vi "StructureFactory.vi"(8 "error in":errorcluster, 11 "reference":refnum<vi>) -> (0 "error out":errorcluster, 3 "structure out":refnum<class "Structure.lvclass">)   [LabVIEW 2014, in "Raspberry Pi Compatible Compiler for LabVIEW.lvlib" / "Structure.lvclass"]
uses:
  Structure.lvclass
  CaseStructure/CaseStructure.lvclass
  Loop/Loop.lvclass
  DiagramDisable/DiagramDisable.lvclass
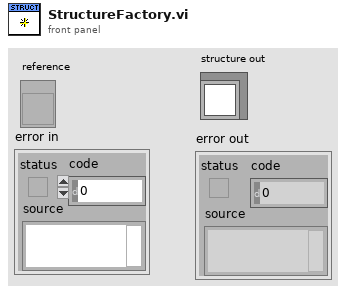
[diagram p1: front panel]
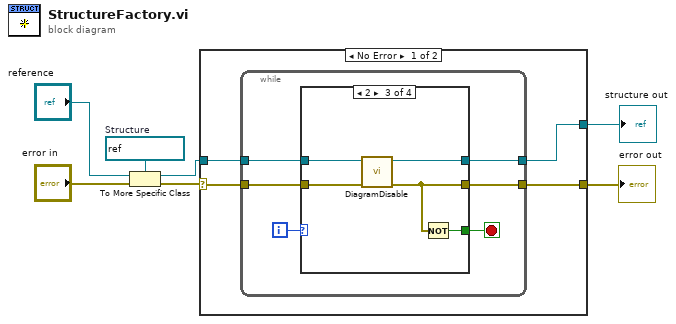
[diagram p0: block diagram]
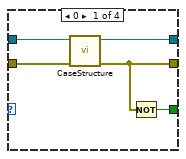
[diagram p2: hidden frame]
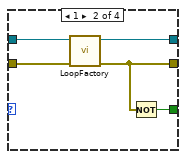
[diagram p3: hidden frame]
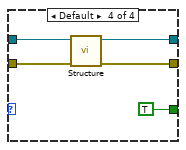
[diagram p4: hidden frame]
diagram:
  w7 = refnum<vi> refnum  # Structure
  n1 = To More Specific Class(target class=w7, reference="reference", error in="error in") -> (specific class reference=w2:refnum<vi>, error out=w1:errorcluster)
  n2 = case shown="No Error" w1 {
    selector: w1 -> [w10 w38]
    tunnel: [w9 _] -> w4
    tunnel: [w8 w38] -> w3
    tunnel: w2 -> [w11 _]
    frame No Error {
      n3 = while {
        tunnel: w10 -> [w16]
        tunnel: [w15] -> w8
        tunnel: [w14] -> w9
        tunnel: w11 -> [w12]
        i -> [w17]
        stop <- w13 stop-if-true
        n4 = case shown="2" w17 {
          tunnel: w16 -> [w21 w26 w31 w36]
          tunnel: [w18 w23 w28 w35] -> w15
          tunnel: [w19 w24 w29 w34] -> w14
          tunnel: [w22 w27 w32 TRUE] -> w13
          tunnel: w12 -> [w20 w25 w30 w33]
          frame 0 {
            n5 = call "CaseStructure.vi"("error in"=w21, "reference"=w20) -> ("error out"=w18:errorcluster, "CaseStructure out"=w19:refnum<class "CaseStructure.lvclass">)  [unwired: 8 in]
            n6 = Not(x=w18) -> (.not. x?=w22:bool)
          }
          frame 1 {
            n7 = call "LoopFactory.vi"("error in"=w26, "reference"=w25) -> ("error out"=w23:errorcluster, "Loop out"=w24:refnum<class "Loop.lvclass">)  [unwired: 8 in]
            n8 = Not(x=w23) -> (.not. x?=w27:bool)
          }
          frame 2 {
            n9 = call "DiagramDisable.vi"("error in"=w31, "reference"=w30) -> ("error out"=w28:errorcluster, "DDS out"=w29:refnum<class "DiagramDisable.lvclass">)  [unwired: 8 in]
            n10 = Not(x=w28) -> (.not. x?=w32:bool)
          }
          frame Default {
            n11 = call "Structure.vi"("error in"=w36, "reference"=w33) -> ("error out"=w35:errorcluster, "structure out"=w34:refnum<class "Structure.lvclass">)  [unwired: 8 in]
          }
        }
      }
    }
    frame Error {
    }
  }
  "error out" <- w3
  "structure out" <- w4
